vi "Key press to move.vi"(0 "keys pressed":T1(array[ring])) -> (1 "move":cluster{"X":dbl, "Y":dbl, "degree":dbl})   [LabVIEW 2019]
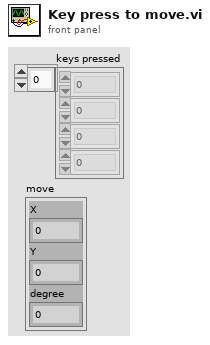
[diagram p1: front panel]
types:
  T1 = enum16{"0", "1", "2", "3", "4", "5", "6", "7", "8", "9", "A", "B", "C", "D", "E", "F", "G", "H", "I", "J", "K", "L", "M", "N", "O", "P", "Q", "R", "S", "T", "U", "V", "W", "X", "Y", "Z", "F1", "F2", "F3", "F4", "F5", "F6", "F7", "F8", "F9", "F10", "F11", "F12", "F13", "F14", "F15", "ADD", "BACK", "BACKSLASH", "CAPITAL", "COMMA", "DECIMAL", "DELETE", "DIVIDE", "DOWN", "END", "EQUALS", "ESCAPE", "GRAVE (`)", "HOME", "INSERT", "LBRACKET", "LCONTROL", "LEFT", "L ALT", "LSHIFT", "LWIN", "MINUS", "MULTIPLY", "NEXT", "NUMLOCK", "NUMPAD_0", "NUMPAD_1", "NUMPAD_2", "NUMPAD_3", "NUMPAD_4", "NUMPAD_5", "NUMPAD_6", "NUMPAD_7", "NUMPAD_8", "NUMPAD_9", "PAUSE", "PERIOD", "PRIOR (PG UP)", "RBRACKET", "RCONTROL", "RETURN", "RIGHT", "R ALT", "RSHIFT", "RWIN", "SCROLL", "SEMICOLON", "SLASH", "SPACE", "SUBTRACT", "TAB", "UP", "ENTER (num pad)", "' (quote)"}[]
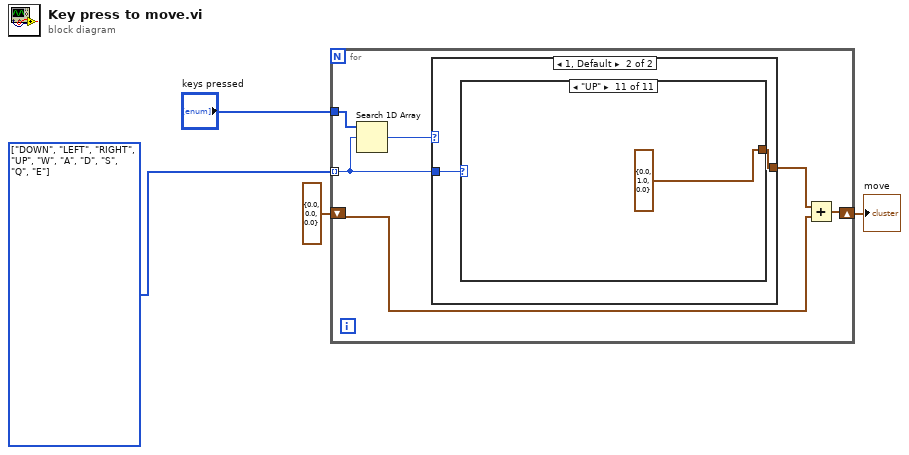
[diagram p0: block diagram]
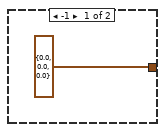
[diagram p2: hidden frame]
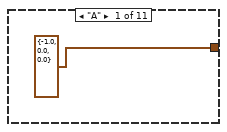
[diagram p3: hidden frame]
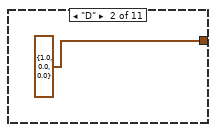
[diagram p4: hidden frame]
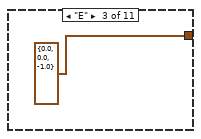
[diagram p5: hidden frame]
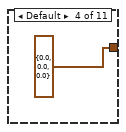
[diagram p6: hidden frame]
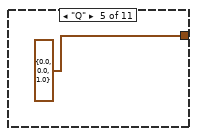
[diagram p7: hidden frame]
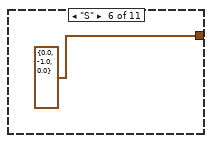
[diagram p8: hidden frame]
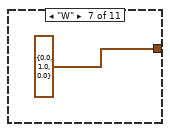
[diagram p9: hidden frame]
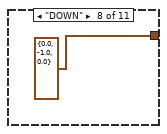
[diagram p10: hidden frame]
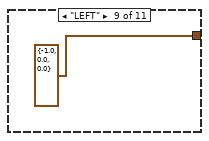
[diagram p11: hidden frame]
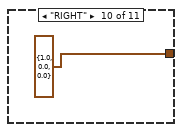
[diagram p12: hidden frame]
diagram:
  w3 = T1 [enum."DOWN", enum."LEFT", enum."RIGHT", enum."UP", enum."W", enum."A", enum."D", enum."S", enum."Q", enum."E"] items=["0", "1", "2", "3", "4", "5", "6", "7", "8", "9", "A", "B", "C", "D", "E", "F", "G", "H", "I", "J", "K", "L", "M", "N", "O", "P", "Q", "R", "S", "T", "U", "V", "W", "X", "Y", "Z", "F1", "F2", "F3", "F4", "F5", "F6", "F7", "F8", "F9", "F10", "F11", "F12", "F13", "F14", "F15", "ADD", "BACK", "BACKSLASH", "CAPITAL", "COMMA", "DECIMAL", "DELETE", "DIVIDE", "DOWN", "END", "EQUALS", "ESCAPE", "GRAVE (`)", "HOME", "INSERT", "LBRACKET", "LCONTROL", "LEFT", "L ALT", "LSHIFT", "LWIN", "MINUS", "MULTIPLY", "NEXT", "NUMLOCK", "NUMPAD_0", "NUMPAD_1", "NUMPAD_2", "NUMPAD_3", "NUMPAD_4", "NUMPAD_5", "NUMPAD_6", "NUMPAD_7", "NUMPAD_8", "NUMPAD_9", "PAUSE", "PERIOD", "PRIOR (PG UP)", "RBRACKET", "RCONTROL", "RETURN", "RIGHT", "R ALT", "RSHIFT", "RWIN", "SCROLL", "SEMICOLON", "SLASH", "SPACE", "SUBTRACT", "TAB", "UP", "ENTER (num pad)", "' (quote)"] ("keys pressed")
  n1 = for {
    tunnel: "keys pressed" -> [w10]
    tunnel: w3 -> [w8] mode=indexing
    shift-right: [w7] -> w1
    shift-left: cluster{"X":dbl, "Y":dbl, "degree":dbl} {"X"=0.0, "Y"=0.0, "degree"=0.0} -> [w5]
    n2 = Search 1D Array(1D array=w10, element=w8) -> (index of element=w9:i32)  [unwired: 1 in]
    n3 = case shown="1, Default" w9 {
      tunnel: w8 -> [_ w13]
      tunnel: [cluster{"X":dbl, "Y":dbl, "degree":dbl} {"X"=0.0, "Y"=0.0, "degree"=0.0} ("robot position") w12] -> w6
      frame -1 {
      }
      frame 1, Default {
        n4 = case shown="\"UP\"" w13 {
          tunnel: [cluster{"X":dbl, "Y":dbl, "degree":dbl} {"X"=-1.0, "Y"=0.0, "degree"=0.0} cluster{"X":dbl, "Y":dbl, "degree":dbl} {"X"=1.0, "Y"=0.0, "degree"=0.0} cluster{"X":dbl, "Y":dbl, "degree":dbl} {"X"=0.0, "Y"=0.0, "degree"=-1.0} cluster{"X":dbl, "Y":dbl, "degree":dbl} {"X"=0.0, "Y"=0.0, "degree"=0.0} ("robot position") cluster{"X":dbl, "Y":dbl, "degree":dbl} {"X"=0.0, "Y"=0.0, "degree"=1.0} cluster{"X":dbl, "Y":dbl, "degree":dbl} {"X"=0.0, "Y"=-1.0, "degree"=0.0} cluster{"X":dbl, "Y":dbl, "degree":dbl} {"X"=0.0, "Y"=1.0, "degree"=0.0} ("robot position") cluster{"X":dbl, "Y":dbl, "degree":dbl} {"X"=0.0, "Y"=-1.0, "degree"=0.0} cluster{"X":dbl, "Y":dbl, "degree":dbl} {"X"=-1.0, "Y"=0.0, "degree"=0.0} cluster{"X":dbl, "Y":dbl, "degree":dbl} {"X"=1.0, "Y"=0.0, "degree"=0.0} cluster{"X":dbl, "Y":dbl, "degree":dbl} {"X"=0.0, "Y"=1.0, "degree"=0.0}] -> w12
          frame "A" {
          }
          frame "D" {
          }
          frame "E" {
          }
          frame Default {
          }
          frame "Q" {
          }
          frame "S" {
          }
          frame "W" {
          }
          frame "DOWN" {
          }
          frame "LEFT" {
          }
          frame "RIGHT" {
          }
          frame "UP" {
          }
        }
      }
    }
    n5 = Add(x=w6, y=w5) -> (x+y=w7:cluster{"X":dbl, "Y":dbl, "degree":dbl})
  }
  "move" <- w1
